vi "integrated-serial-read.vi"() -> ()   [LabVIEW 2021]
uses:
  <vilib>/Instr/_visa.llb/VISA Configure Serial Port (Instr).vi
  <vilib>/regexp/Match Regular Expression.xnode
panel:
  out "RHT6: Humidity (%)":dbl format="%.2f"
  out "RHT6: Temp (degC)":dbl format="%.2f"
  out "RHT5: Humidity (%)":dbl format="%.2f"
  out "RHT5: Temp (degC)":dbl format="%.2f"
  out "RHT4: Humidity (%)":dbl format="%.2f"
  out "RHT4: Temp (degC)":dbl format="%.2f"
  out "RHT3: Humidity (%)":dbl format="%.2f"
  out "RHT3: Temp (degC)":dbl format="%.2f"
  out "CD6: CO2 (ppm)":dbl format="%.2f"
  out "CD5: CO2 (ppm)":dbl format="%.2f"
  out "CD4: CO2 (ppm)":dbl format="%.2f"
  out "CD3: CO2 (ppm)":dbl format="%.2f"
  out "CD2: Humidity (%)":dbl format="%.2f"
  out "CD2: Temp (degC)":dbl format="%.2f"
  out "CD2: CO2 (ppm)":dbl format="%.2f"
  out "Num Samples":i32
  out "error out":errorcluster
  out "CD1: Humidity (%)":dbl format="%.2f"
  out "CD1: Temp (degC)":dbl format="%.2f"
  out "CD1: CO2 (ppm)":dbl format="%.2f"
  out "data string array":string[](array[string])
  in  "Stop Button":bool
  out "read buffer":string
  out "Bytes Returned":u32
  in  "VISA resource name":refnum<visa-resource-name>="COM22"
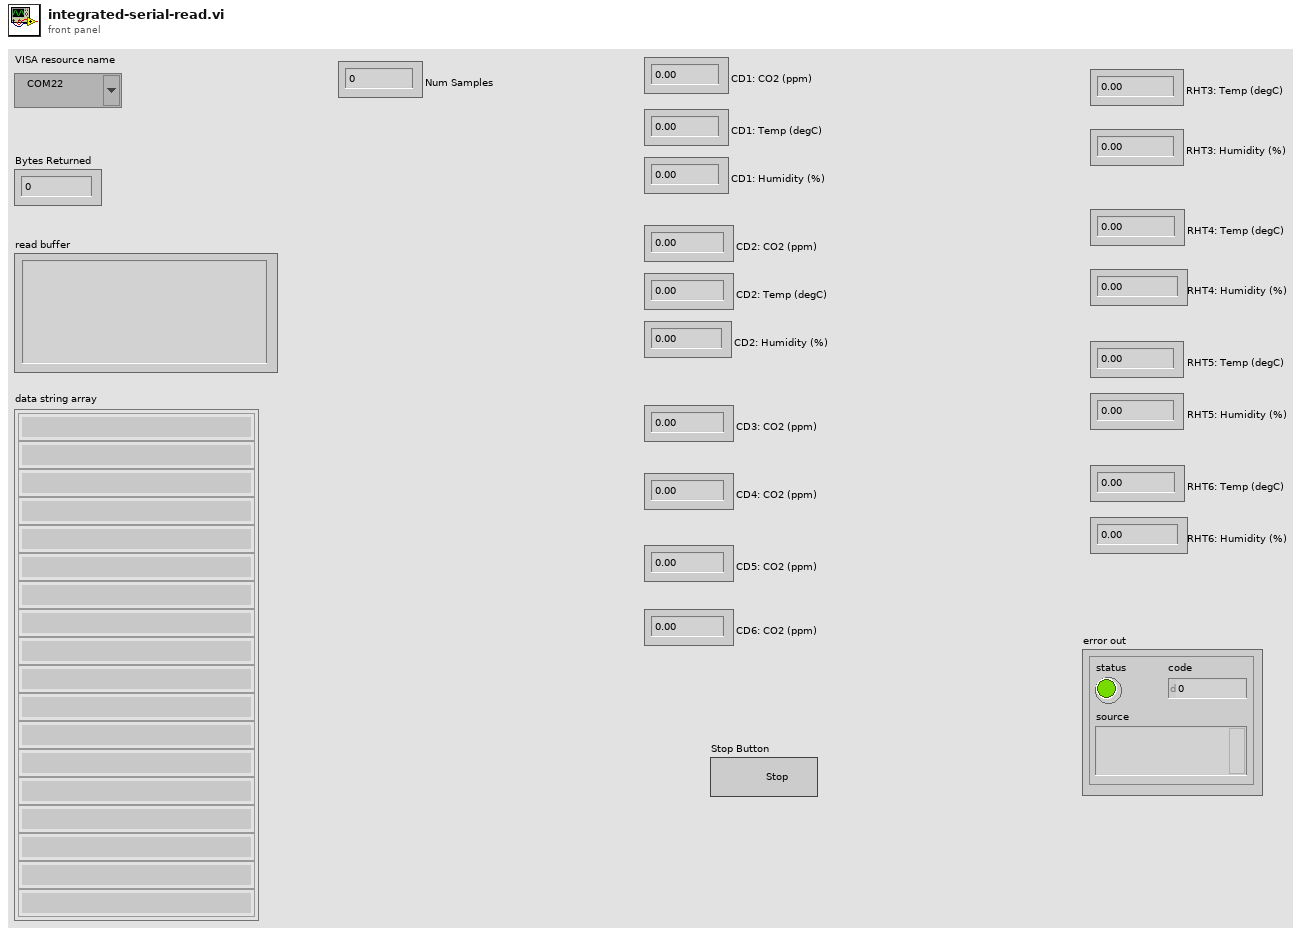
[diagram p1: front panel]
types:
  T1 = typedef "SCD41.ctl" = cluster{"CO2 (ppm)":dbl, "Temp (degC)":dbl, "Humidity (%)":dbl}
  T2 = typedef "STC31.ctl" = cluster{"CO2 (ppm)":dbl}
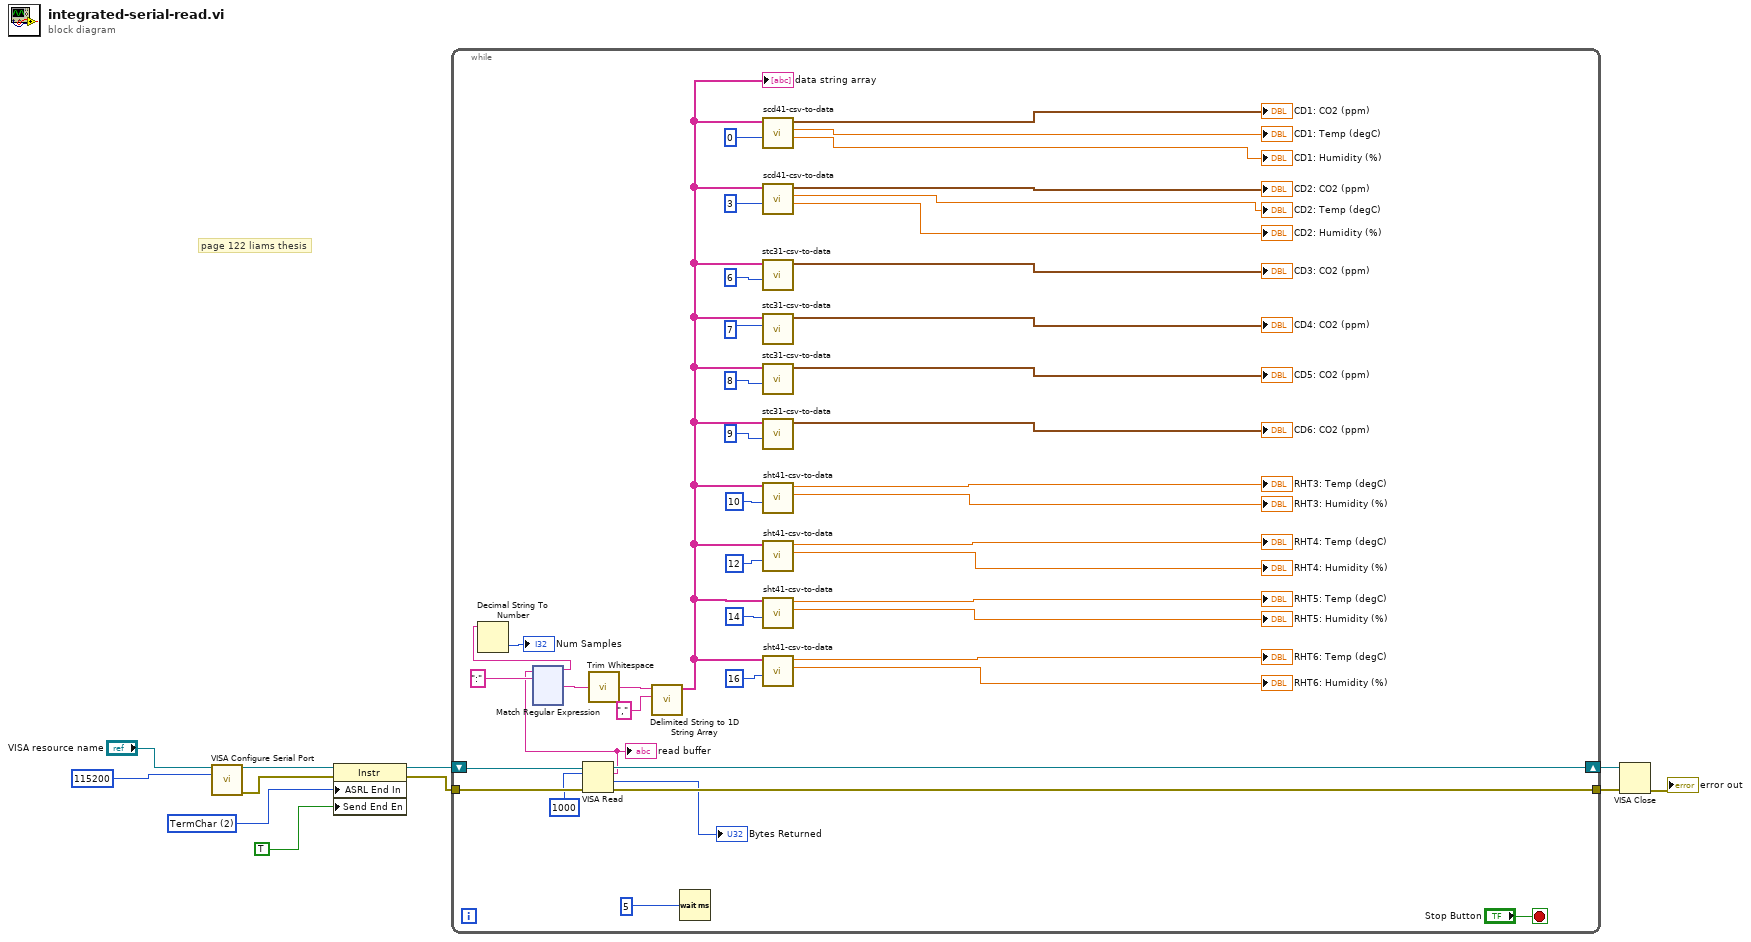
[diagram p0: block diagram]
diagram:
  w7 = u16 2 items=["None", "Last Bit", "TermChar"] ("Serial Settings:End Mode for Reads")
  # "page 122 liams thesis"
  n1 = call-poly "VISA Configure Serial Port"("VISA resource name"="VISA resource name", "baud rate (9600)"=u32 115200) -> ("VISA resource name out"=w9:refnum<visa-resource-name>, "error out"=w8:errorcluster)  [unwired: 12 in]
  n2 = property class="Instr"(reference=w9, error in=w8, "ASRL End In"=w7, "Send End En"=TRUE ("Message Based Settings:Send End Enable")) -> (reference out=w5:refnum<visa-resource-name>, error out=w4:errorcluster)
  n3 = while {
    tunnel: w4 -> [w53]
    shift-right: [w50] -> w2
    shift-left: w5 -> [w55]
    tunnel: [w51] -> w3
    stop <- "Stop Button" stop-if-true
    n4 = VISA Read(VISA resource name=w55, byte count=u32 1000, error in (no error)=w53) -> (VISA resource name out=w50:refnum<visa-resource-name>, read buffer=w45:string, return count=→"Bytes Returned":u32, error out=w51:errorcluster)
    "read buffer" <- w45
    n5 = xnode "Match Regular Expression"("input string"=w45, "regular expression"=":" ("delimiter")) -> ("before match"=w44:string, "after match"=w42:string)  [unwired: 4 in, 3 out]
    n6 = Decimal String To Number(string=w44) -> (number=→"Num Samples":i32)  [unwired: 2 in, 1 out]
    n7 = call <vilib>:"Trim Whitespace.vi"("string"=w42) -> ("trimmed string"=w41:string)  [unwired: 1 in]
    n8 = call <vilib>:"Delimited String to 1D String Array.vi"("delimiter"=",", "delimited string"=w41) -> ("string array"=w13:string[])  [unwired: 9 in]
    "data string array" <- w13
    n9 = Wait (ms)(milliseconds to wait=u32 5) -> ()  [unwired: 1 out]
    n10 = call "scd41-csv-to-data.vi"(9:0 ("Starting Index"), "sensor-csv-input"=w13) -> ("SCD41: Temp (degC)"=→"CD1: Humidity (%)":dbl, "SCD41: CO2 (ppm)"=→"CD1: Temp (degC)":dbl, "SCD typedef"=→"CD1: CO2 (ppm)":T1)  [unwired: 6 in, 1 out]
    n11 = call "scd41-csv-to-data.vi"(9:3 ("Starting Index"), "sensor-csv-input"=w13) -> ("SCD41: Temp (degC)"=→"CD2: Humidity (%)":dbl, "SCD41: CO2 (ppm)"=→"CD2: Temp (degC)":dbl, "SCD typedef"=→"CD2: CO2 (ppm)":T1)  [unwired: 6 in, 1 out]
    n12 = call "stc31-csv-to-data.vi"(9:6 ("index"), "sensor-csv-input"=w13) -> ("STC31: data output"=→"CD3: CO2 (ppm)":T2)  [unwired: 7 in, 2 out]
    n13 = call "stc31-csv-to-data.vi"(9:7 ("Starting Index"), "sensor-csv-input"=w13) -> ("STC31: data output"=→"CD4: CO2 (ppm)":T2)  [unwired: 7 in, 2 out]
    n14 = call "stc31-csv-to-data.vi"(9:8 ("Starting Index"), "sensor-csv-input"=w13) -> ("STC31: data output"=→"CD5: CO2 (ppm)":T2)  [unwired: 7 in, 2 out]
    n15 = call "stc31-csv-to-data.vi"(9:9 ("Starting Index"), "sensor-csv-input"=w13) -> ("STC31: data output"=→"CD6: CO2 (ppm)":T2)  [unwired: 7 in, 2 out]
    n16 = call "sht41-csv-to-data.vi"("Starting Index"=10, "Data In (string array)"=w13) -> ("SHT41: Humidity (%)"=→"RHT3: Humidity (%)":dbl, "SHT41: Temp (degC)"=→"RHT3: Temp (degC)":dbl)  [unwired: 7 in, 1 out]
    n17 = call "sht41-csv-to-data.vi"("Starting Index"=12, "Data In (string array)"=w13) -> ("SHT41: Humidity (%)"=→"RHT4: Humidity (%)":dbl, "SHT41: Temp (degC)"=→"RHT4: Temp (degC)":dbl)  [unwired: 7 in, 1 out]
    n18 = call "sht41-csv-to-data.vi"("Starting Index"=14, "Data In (string array)"=w13) -> ("SHT41: Humidity (%)"=→"RHT5: Humidity (%)":dbl, "SHT41: Temp (degC)"=→"RHT5: Temp (degC)":dbl)  [unwired: 7 in, 1 out]
    n19 = call "sht41-csv-to-data.vi"("Starting Index"=16, "Data In (string array)"=w13) -> ("SHT41: Humidity (%)"=→"RHT6: Humidity (%)":dbl, "SHT41: Temp (degC)"=→"RHT6: Temp (degC)":dbl)  [unwired: 7 in, 1 out]
  }
  n20 = VISA Close(VISA resource name=w2, error in (no error)=w3) -> (error out=→"error out":errorcluster)
